vi "Actor Core.vi"(8 "error in":errorcluster, 11 "Orphan Detector in":refnum<class "Orphan Detector.lvclass">) -> (0 "error out":errorcluster, 3 "Actor out":refnum<class "Actor.lvclass">)   [LabVIEW 2023, in "Monitored Actor.lvlib" / "Orphan Detector.lvclass"]
doc: "(<B>Filename</B>: Actor Framework.lvlib:Actor.lvclass:Actor Core.vi)\n\nReceives messages to the actor, reacts to them, and initiates any error handling that may shut the actor down.\n\nDescendant classes may override this VI to append parallel tasks for the actor to complete while it handles messages. Overrides use the Call Parent Method node."
uses:
  Orphan Detector.lvclass
  builds/Framework/Actor Framework.lvlibp/1abvi3w/vi.lib/ActorFramework/Actor/Actor.lvclass
  Monitor Data/Actor Data.ctl
  builds/Framework/Actor Framework.lvlibp/1abvi3w/vi.lib/ActorFramework/Message Enqueuer/Message Enqueuer.lvclass
  Orphan Detector.lvclass/Orphan Detector.ctl
  <vilib>/Utility/miscctls.llb/LVRowAndColumnTypeDef.ctl
  builds/Framework/Actor Framework.lvlibp/1abvi3w/vi.lib/ActorFramework/Message/Message.lvclass
  Monitor Data/Monitor Data.lvclass
panel:
  in  "Poll Rate":i32=500 caption="ms"
  in  "Orphans":i32(listbox)
  # "Orphans"
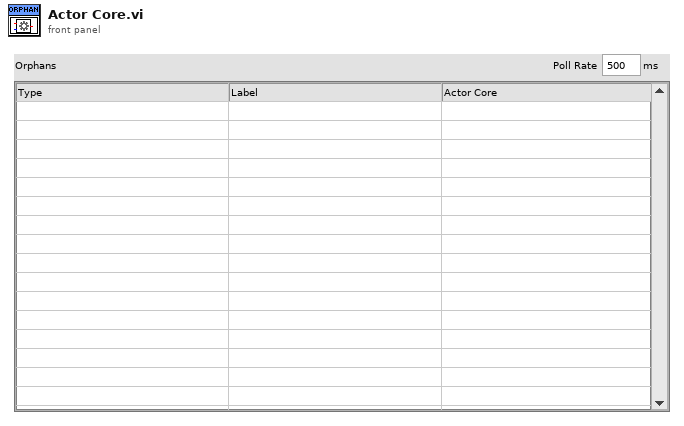
[diagram p1: front panel]
types:
  T1 = enum32{"Invalid", "Standard", "Closed", "Hidden", "Minimized", "Maximized"}
  T2 = typedef "Monitored Actor.lvlib/Monitor Data.lvclass/Actor Data.ctl" = cluster{"Actor Type":string, "Actor Core VI":string, "Self":refnum<class "Message Enqueuer.lvclass">, "Caller":refnum<class "Message Enqueuer.lvclass">, "Actor Label":string, "Last Ping":dbl}
  T3 = typedef "LVRowAndColumnTypeDef.ctl" = cluster{"Row":i32, "Column":i32}
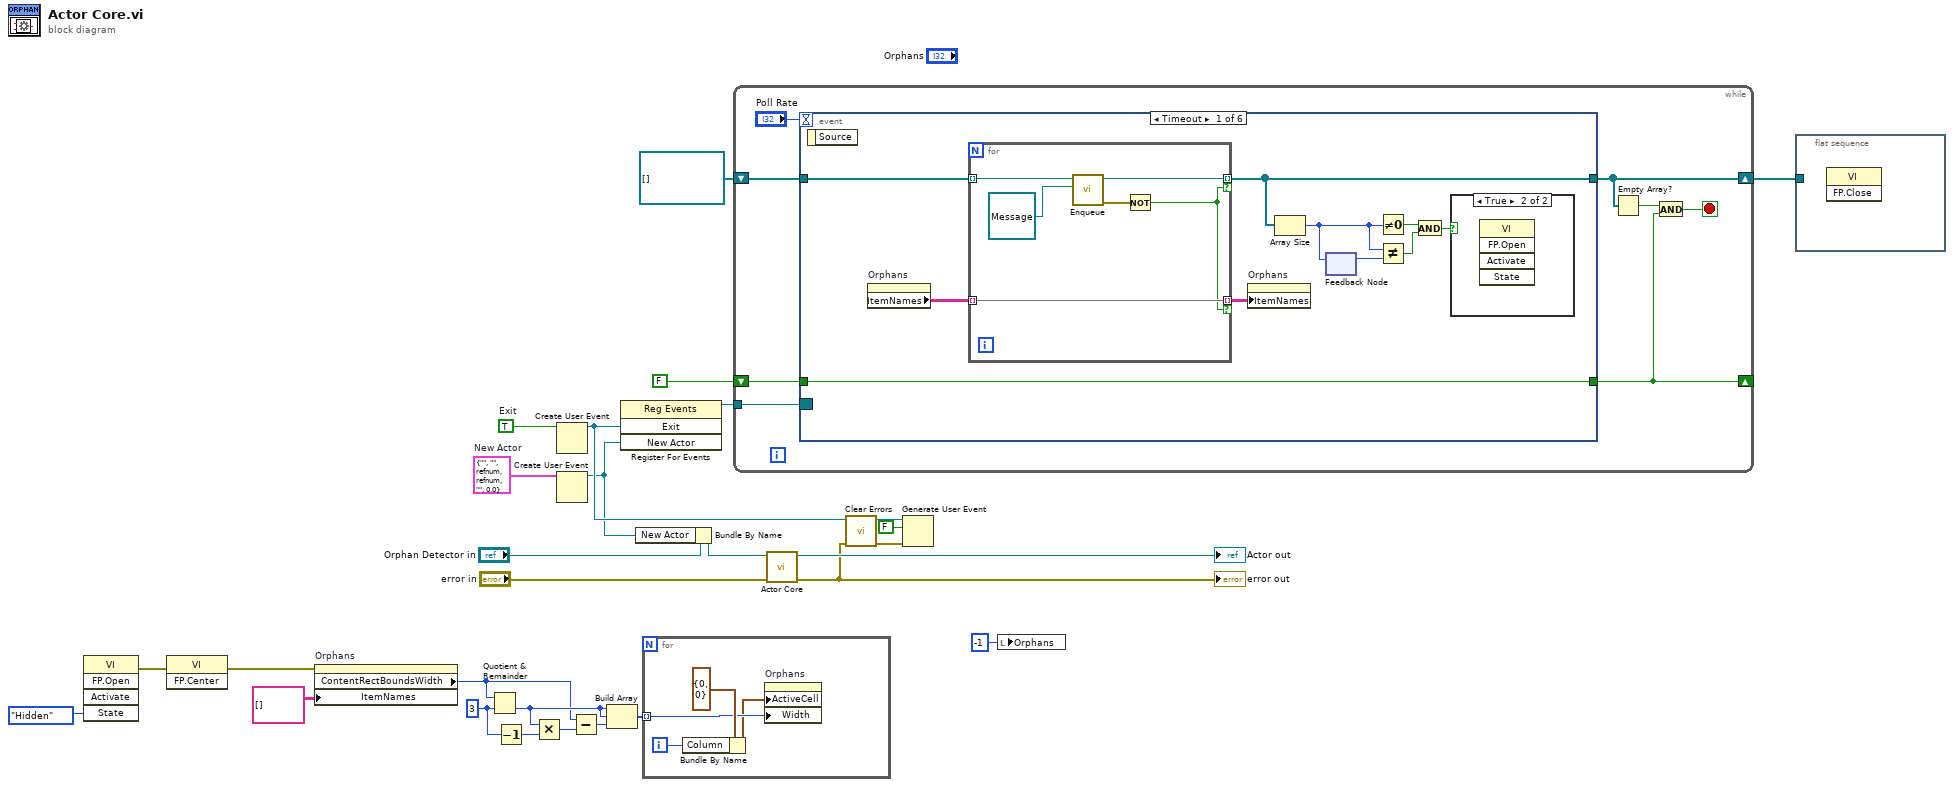
[diagram p0: block diagram]
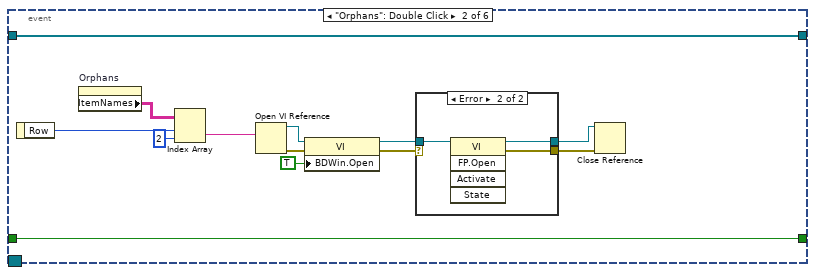
[diagram p3: hidden frame]
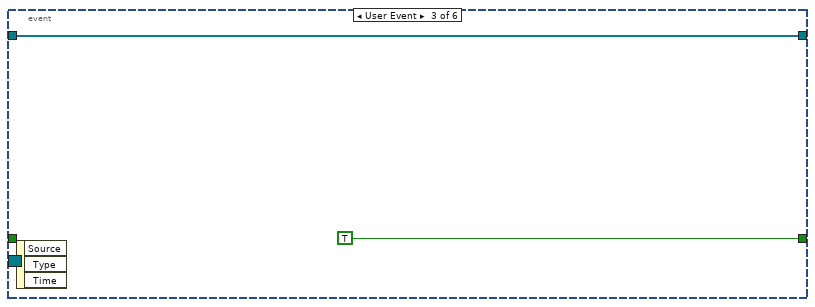
[diagram p5: hidden frame]
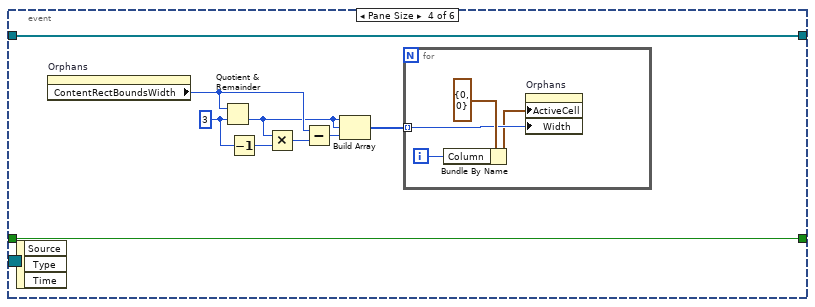
[diagram p6: hidden frame]
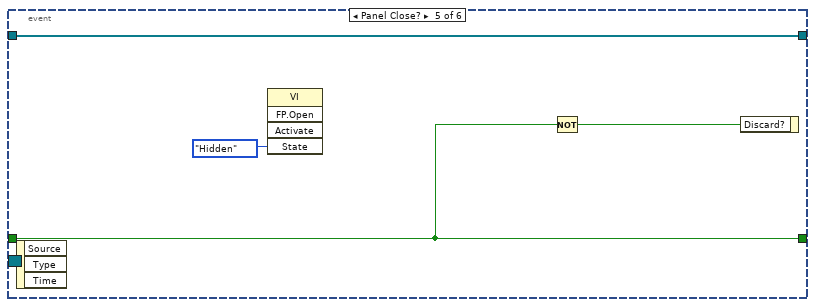
[diagram p7: hidden frame]
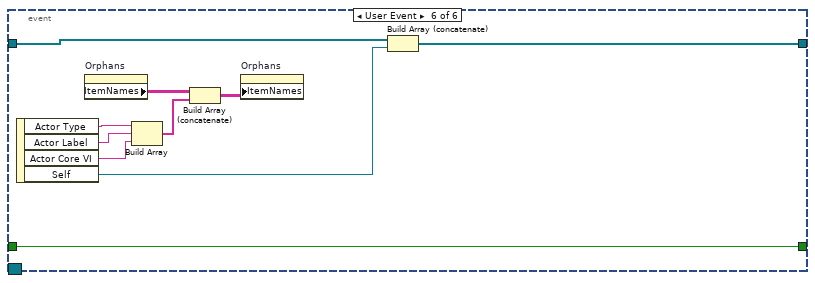
[diagram p8: hidden frame]
diagram:
  w17 = TRUE  # Exit
  w11 = T2 {"Actor Type"="", "Actor Core VI"="", "Self"=refnum, "Caller"=refnum, "Actor Label"="", "Last Ping"=0.0}  # New Actor
  w23 = 3 ("y")
  n1 = invoke class="VI" method="FP.Open"("State"=T1."Hidden") -> (error out=w6:errorcluster)  [unwired: 4 in, 4 out]
  n2 = invoke class="VI" method="FP.Center"(error in=w6) -> (error out=w5:errorcluster)  [unwired: 2 in, 2 out]
  n3 = property on="Orphans" class="MCListbox (strict)"(error in=w5, "ItemNames"=string[][] [] ("Item Names")) -> ("ContentRectBoundsWidth"=w18:i32)  [unwired: 1 in, 2 out]
  n4 = Quotient & Remainder(x=w18, y=w23) -> (floor(x/y)=w19:i32)  [unwired: 1 out]
  n5 = Decrement(x=w23) -> (x-1=w22:i32)
  n6 = Multiply(x=w19, y=w22) -> (x*y=w20:i32)
  n7 = Create User Event(user event datatype=w17) -> (user event=w13:refnum<user-event>)  [unwired: 1 in, 1 out]
  n8 = Create User Event(user event datatype=w11) -> (user event=w1:refnum<user-event>)  [unwired: 1 in, 1 out]
  n9 = Subtract(x=w18, y=w20) -> (x-y=w24:i32)
  n10 = Build Array(w19, w19, w24) -> (w21:i32[])
  n11 = register-events(w13, w1) -> (reference out=w16:refnum<event-registration>)  [unwired: 2 in, 1 out]
  n12 = Bundle By Name(cluster="Orphan Detector in", "New Actor"=w1) -> (w10:refnum<class "Orphan Detector.lvclass">)
  n13 = for {
    tunnel: w21 -> [w30] mode=indexing
    i -> [w28]
    n14 = Bundle By Name(cluster=T3 {"Row"=0, "Column"=0} ("Active Cell:Active Cell"), "Column"=w28) -> (w29:T3)
    n15 = property on="Orphans" class="MCListbox (strict)"("ActiveCell"=w29, "Width"=w30) -> ()  [unwired: 2 in, 2 out]
  }
  n16 = while {
    tunnel: w16 -> [w39]
    shift-right: [w35] -> w3
    shift-left: refnum<class "Message Enqueuer.lvclass">[] [] -> [w37]
    shift-right: [w33] -> _
    shift-left: FALSE -> [w36]
    stop <- w32 stop-if-true
    n17 = event shown="[0] Timeout" {
      selector: w39 -> [_ _ _ _ _ _]
      dyn-events: _ -> [_ _ _ _ _ _]
      timeout: "Poll Rate" -> [_ _ _ _ _ _]
      tunnel: [w46 w68 w75 w77 w92 w95] -> w35
      tunnel: w37 -> [w49 w68 w75 w77 w92 w94]
      tunnel: [w40 w64 TRUE w76 w90 w93] -> w33
      tunnel: w36 -> [w40 w64 _ w76 w90 w93]
      event Timeout {
        n18 = event-data() -> ()  [unwired: 1 in, 1 out]
        n19 = property on="Orphans" class="MCListbox (strict)"() -> ("ItemNames"=w48:string[][])  [unwired: 2 in, 2 out]
        n20 = for {
          tunnel: w49 -> [w55] mode=indexing
          tunnel: w48 -> [w52] mode=indexing
          tunnel: [w53] -> w46 mode=indexing if=w50
          tunnel: [w52] -> w47 mode=indexing if=w50
          n21 = call "Enqueue.vi"("Message"=refnum<class "Message.lvclass"> refnum, "Message Enqueuer in"=w55) -> ("error out"=w51:errorcluster, "Message Enqueuer out"=w53:refnum<class "Message Enqueuer.lvclass">)  [unwired: 8 in]
          n22 = Not(x=w51) -> (.not. x?=w50:bool)
        }
        n23 = property on="Orphans" class="MCListbox (strict)"("ItemNames"=w47) -> ()  [unwired: 2 in, 2 out]
        n24 = Array Size(array=w46) -> (size(s)=w44:i32)
        n25 = feedback-in #1(w44) -> ()
        n26 = feedback #1() -> (w45:i32)  [unwired: 1 in]
        n27 = Not Equal To 0?(x=w44) -> (x != 0?=w43:bool)
        n28 = Not Equal?(x=w44, y=w45) -> (x != y?=w42:bool)
        n29 = And(x=w43, y=w42) -> (x .and. y?=w41:bool)
        n30 = case shown="True" w41 {
          frame False {
          }
          frame True {
            n31 = invoke class="VI" method="FP.Open"() -> ()  [unwired: 5 in, 5 out]
          }
        }
      }
      event "Orphans": Double Click {
        n32 = event-data() -> ("Row"=w66:i32)  [unwired: 1 in]
        n33 = property on="Orphans" class="MCListbox (strict)"() -> ("ItemNames"=w67:string[][])  [unwired: 2 in, 2 out]
        n34 = Index Array(array=w67, index (row)=w66, index (col)=2 ("disabled index (col)")) -> (element=w56:string)
        n35 = Open VI Reference(vi path=w56) -> (vi reference=w63:refnum<vi>, error out=w62:errorcluster)  [unwired: 5 in]
        n36 = property class="VI"(reference=w63, error in=w62, "BDWin.Open"=TRUE ("Block Diagram Window:Open")) -> (reference out=w61:refnum<vi>, error out=w60:errorcluster)
        n37 = case shown="Error" w60 {
          selector: w60 -> [w70 _]
          tunnel: w61 -> [w69 w73]
          tunnel: [w69 w72] -> w57
          tunnel: [w70 w71] -> w58
          frame No Error {
          }
          frame Error {
            n38 = invoke class="VI" method="FP.Open"(reference=w73) -> (reference out=w72:refnum<vi>, error out=w71:errorcluster)  [unwired: 4 in, 3 out]
          }
        }
        n39 = Close Reference(reference=w57, error in (no error)=w58) -> ()  [unwired: 1 out]
      }
      event User Event {
        n40 = event-data() -> ()  [unwired: 1 in, 3 out]
      }
      event Pane Size {
        w79 = 3 ("y")
        n41 = event-data() -> ()  [unwired: 1 in, 3 out]
        n42 = property on="Orphans" class="MCListbox (strict)"() -> ("ContentRectBoundsWidth"=w84:i32)  [unwired: 2 in, 2 out]
        n43 = Quotient & Remainder(x=w84, y=w79) -> (floor(x/y)=w83:i32)  [unwired: 1 out]
        n44 = Decrement(x=w79) -> (x-1=w80:i32)
        n45 = Multiply(x=w83, y=w80) -> (x*y=w82:i32)
        n46 = Subtract(x=w84, y=w82) -> (x-y=w78:i32)
        n47 = Build Array(w83, w83, w78) -> (w81:i32[])
        n48 = for {
          tunnel: w81 -> [w87] mode=indexing
          i -> [w85]
          n49 = Bundle By Name(cluster=T3 {"Row"=0, "Column"=0} ("Active Cell:Active Cell"), "Column"=w85) -> (w86:T3)
          n50 = property on="Orphans" class="MCListbox (strict)"("ActiveCell"=w86, "Width"=w87) -> ()  [unwired: 2 in, 2 out]
        }
      }
      event Panel Close? {
        n51 = event-data() -> ()  [unwired: 1 in, 3 out]
        n52 = invoke class="VI" method="FP.Open"("State"=T1."Hidden") -> ()  [unwired: 4 in, 5 out]
        n53 = Not(x=w90) -> (.not. x?=w89:bool)
        n54 = event-data("Discard?"=w89) -> ()  [unwired: 1 in, 1 out]
      }
      event User Event {
        n55 = event-data() -> ("Actor Type"=w102:string, "Actor Label"=w101:string, "Actor Core VI"=w100:string, "Self"=w96:refnum<class "Message Enqueuer.lvclass">)  [unwired: 1 in]
        n56 = property on="Orphans" class="MCListbox (strict)"() -> ("ItemNames"=w99:string[][])  [unwired: 2 in, 2 out]
        n57 = Build Array(w102, w101, w100) -> (w97:string[])
        n58 = Build Array (concatenate)(w99, w97) -> (w98:string[][])
        n59 = property on="Orphans" class="MCListbox (strict)"("ItemNames"=w98) -> ()  [unwired: 2 in, 2 out]
        n60 = Build Array (concatenate)(w94, w96) -> (w95:refnum<class "Message Enqueuer.lvclass">[])
      }
    }
    n61 = Empty Array?(array=w35) -> (empty?=w34:bool)
    n62 = And(x=w34, y=w33) -> (x .and. y?=w32:bool)
  }
  n63 = call-parent "Actor Core.vi"("error in"="error in", "Actor in"=w10) -> ("error out"=w15:errorcluster, "Actor out"=→"Actor out":refnum<class "Actor.lvclass">)  [unwired: 8 in]
  "error out" <- w15
  n64 = call <vilib>:"Clear Errors.vi"("error in (no error)"=w15) -> ("error out"=w14:errorcluster)  [unwired: 5 in, 1 out]
  n65 = Generate User Event(user event=w13, event data cluster=FALSE ("event data"), error in=w14) -> ()  [unwired: 1 in, 2 out]
  n66 = local write "Orphans"(-1 ("Orphans")) -> ()
  n67 = flat-sequence {
    tunnel: w3 -> [_]
    frame #0 {
      n68 = invoke class="VI" method="FP.Close"() -> ()  [unwired: 3 in, 3 out]
    }
  }
